vi "FPGA Combined SAR and DSA.vi"() -> ()   [LabVIEW 2025]
uses:
  <vilib>/Platform/TimedLoop/XDataNode/timing_clust.ctl
  <vilib>/Platform/TimedLoop/XDataNode/nitl_modes.ctl
  <vilib>/Platform/TimedLoop/XDataNode/wakeup.ctl
  <vilib>/LabVIEW Targets/FPGA/cRIO/shared/nicrio_ModuleControls/nicrio_cRIO-9234_DataRatesRing2.ctl
  <vilib>/rvi/Emulation/niFpgaGetClockAttributes.vi
  <vilib>/rvi/Emulation/niFpgaSctlEmulationGetInTimedLoop.vi
  <vilib>/rvi/Emulation/niFpgaEmulationReportErrorSimple.vi
  <vilib>/rvi/eio/common/nirviEmuTemplateMethod_errors.vi
  <vilib>/rvi/Emulation/niFpgaCriticalErrorInLSC.vi
  <vilib>/rvi/eio/common/nirviEmuTemplatePropertySet_noerrors.vi
  <vilib>/eio/utilities/niEioResolveVilibRelativePath.vi
  <vilib>/rvi/interface/RandomDataEmulation/niFpgaRandomDataHandleErrors.vi
  <vilib>/eio/EIONode/EIONode.xnode
  <vilib>/eio/EIOPropertyNode/EIOPropertyNode.xnode
  <vilib>/rvi/DataTransferAndStorage/Container/XNode/niFpgaContainer.xnode
  <vilib>/rvi/interface/RandomDataEmulation/nirviRandomDataFpgaReadWriteTemplate.vi
  <vilib>/platform/TimedLoop/XDataNode/XDataNode.xnode
  <vilib>/rvi/eio/common/nirviEmuTemplatePropertyGet_errors.vi
  <vilib>/rvi/eio/common/nirviEmuTemplatePropertyGet_noerrors.vi
  <vilib>/rvi/eio/common/nirviEmuTemplatePropertySet_errors.vi
  <vilib>/Platform/TimedLoop/XDataNode/XDNodeRunTimeDep.lvlib
panel:
  in  "stop Fast Digital":bool
  out "Mod2/DIO0":bool
  out "Mod2/DIO1":bool
  out "Mod2/DIO2":bool
  out "Mod2/DIO3":bool
  in  "stop Slow Digital":bool
  in  "Mod1/DO0":bool
  in  "Mod1/DO1":bool
  in  "Mod1/DO2":bool
  in  "Mod1/DO3":bool
  out "Combined Data":fxp<+/-,26,5>[](array[numeric])
  in  "stop Combined":bool
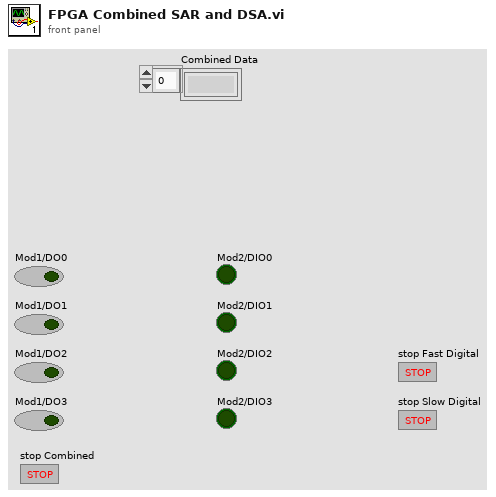
[diagram p1: front panel]
types:
  T1 = typedef "nicrio_cRIO-9234_DataRatesRing2.ctl" = u8
  T2 = typedef "XDNodeRunTimeDep.lvlib/timing_clust.ctl" = cluster{"Expected End [f-1]":u64, "Actual End [f-1]":u64, "Finished Late? [f-1]":bool, "Expected End [i-1]":u64, "Actual End [i-1]":u64, "Finished Late? [i-1]":bool, "Expected Start [i]":u64, "Actual Start [i]":u64, "Expected Start [f]":u64, "Actual Start [f]":u64, "Source Name":string, "Structure Name":string, "Period":i64, "Deadline":i64, "Offset":i64, "Start":i64, "Priority":i32, "Timeout":i32, "Mode":T3, "Wakeup Reason":T4, "Error":errorcluster, "Source Type":string, "Secondary Source Type":string, "Global End Time":u64, "Global Start Time":u64, "Frame Duration":u64, "Iteration Duration":u64, "Assigned CPU":i32, "I/O Scan Engine Mode":u32}
  T3 = typedef "XDNodeRunTimeDep.lvlib/nitl_modes.ctl" = enum32{"No Change", "Process missed periods, maintain original phase", "Discard missed periods, maintain original phase", "Process missed periods, ignore original phase", "Discard missed periods, ignore original phase"}
  T4 = typedef "XDNodeRunTimeDep.lvlib/wakeup.ctl" = enum32{"Normal", "Aborted", "Asynchronous wakeup", "Timing source error", "Timed loop error", "Timeout"}
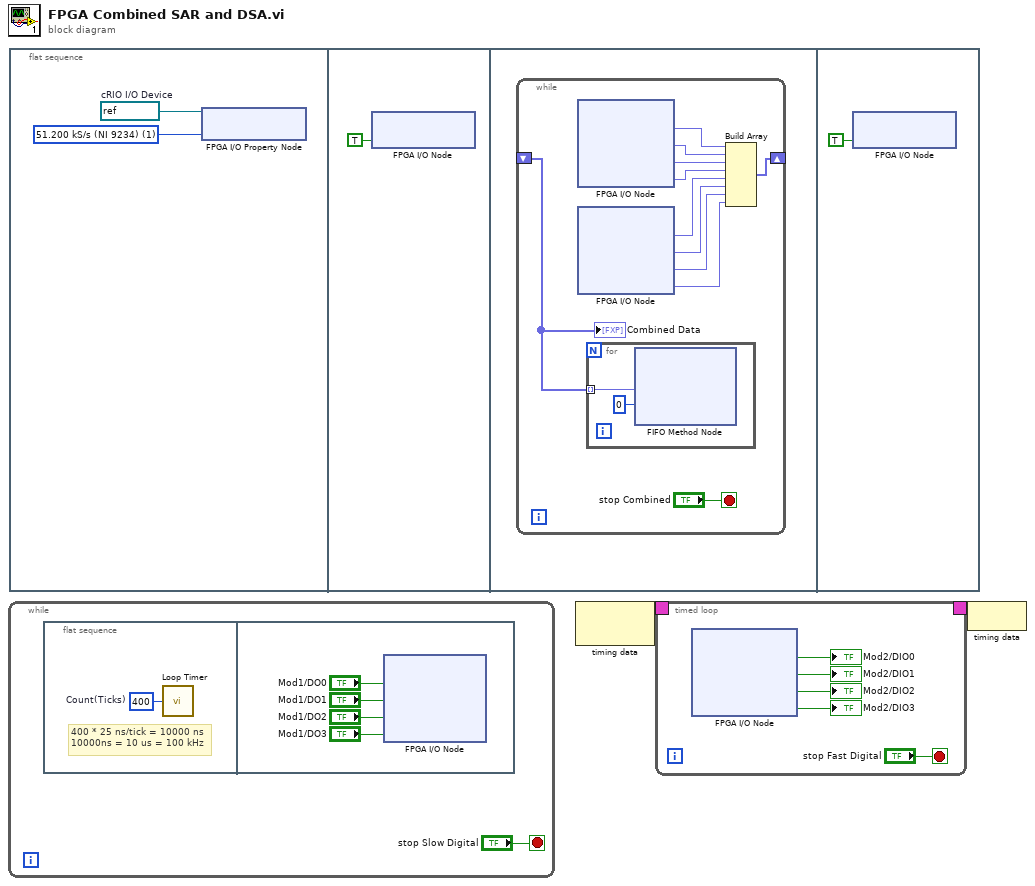
[diagram p0: block diagram]
diagram:
  n1 = while {
    stop <- "stop Slow Digital" stop-if-true
    n2 = flat-sequence {
      frame #0 {
        w4 = u32 400  # Count(Ticks)
        # "400 * 25 ns/tick = 10000 ns\n10000ns = 10 us = 100 kHz"
        n3 = call "Loop Timer"("Count(Ticks)"=w4) -> ()  [unwired: 1 out]
      }
      frame #1 {
        n4 = xnode "FPGA I/O Node"("Mod1/DO0"="Mod1/DO0", "Mod1/DO1"="Mod1/DO1", "Mod1/DO2"="Mod1/DO2", "Mod1/DO3"="Mod1/DO3") -> ()  [unwired: 4 in, 4 out]
      }
    }
  }
  n5 = flat-sequence {
    frame #0 {
      w9 = T1 1 items=["51.200 kS/s (NI 9234)"=1, "25.600 kS/s (NI 9234)"=2, "17.067 kS/s (NI 9234)"=3, "12.800 kS/s (NI 9234)"=4, "10.240 kS/s (NI 9234)"=5, "8.533 kS/s (NI 9234)"=6, "7.314 kS/s (NI 9234)"=7, "6.400 kS/s (NI 9234)"=8, "5.689 kS/s (NI 9234)"=9, "5.120 kS/s (NI 9234)"=10, "4.654 kS/s (NI 9234)"=11, "4.267 kS/s (NI 9234)"=12, "3.938 kS/s (NI 9234)"=13, "3.657 kS/s (NI 9234)"=14, "3.413 kS/s (NI 9234)"=15, "3.200 kS/s (NI 9234)"=16, "3.012 kS/s (NI 9234)"=17, "2.845 kS/s (NI 9234)"=18, "2.695 kS/s (NI 9234)"=19, "2.560 kS/s (NI 9234)"=20, "2.438 kS/s (NI 9234)"=21, "2.328 kS/s (NI 9234)"=22, "2.226 kS/s (NI 9234)"=23, "2.133 kS/s (NI 9234)"=24, "2.048 kS/s (NI 9234)"=25, "1.969 kS/s (NI 9234)"=26, "1.896 kS/s (NI 9234)"=27, "1.829 kS/s (NI 9234)"=28, "1.765 kS/s (NI 9234)"=29, "1.707 kS/s (NI 9234)"=30, "1.652 kS/s (NI 9234)"=31] ("Data Rate")
      w10 = refnum<k21> "Mod7"  # cRIO I/O Device
      n6 = xnode "FPGA I/O Property Node"("FPGA I/O In"=w10, "Data Rate"=w9) -> ()  [unwired: 1 out]
    }
    frame #1 {
      n7 = xnode "FPGA I/O Node"("Mod7/Start"=TRUE) -> ()  [unwired: 1 in, 1 out]
    }
    frame #2 {
      n8 = while {
        shift-right: [w21] -> _
        shift-left: _ -> [w12]
        stop <- "stop Combined" stop-if-true
        n9 = xnode "FPGA I/O Node"() -> ("Mod7/AI0"=w20:fxp<+/-,24,4>, "Mod7/AI1"=w19:fxp<+/-,24,4>, "Mod7/AI2"=w18:fxp<+/-,24,4>, "Mod7/AI3"=w17:fxp<+/-,24,4>)  [unwired: 4 in, 4 out]
        n10 = xnode "FPGA I/O Node"() -> ("Mod4/AI0"=w16:fxp<+/-,26,5>, "Mod4/AI1"=w15:fxp<+/-,26,5>, "Mod4/AI2"=w14:fxp<+/-,26,5>, "Mod4/AI3"=w13:fxp<+/-,26,5>)  [unwired: 4 in, 4 out]
        n11 = for {
          tunnel: w12 -> [w24] mode=indexing
          n12 = xnode ("FIFO Method Node")("Element"=w24, "Timeout"=0) -> ()  [unwired: 1 in, 2 out]
        }
        n13 = Build Array(w20, w19, w18, w17, w16, w15, w14, w13) -> (w21:fxp<+/-,26,5>[])
        "Combined Data" <- w12
      }
    }
    frame #3 {
      n14 = xnode "FPGA I/O Node"("Mod7/Stop"=TRUE ("Mod7/Start")) -> ()  [unwired: 1 in, 1 out]
    }
  }
  n15 = node-c288() -> (w2:T2)  [unwired: 1 in]
  n16 = timed-loop {
    timing: w2 -> [_]
    timing-out: [_] -> w1
    stop <- "stop Fast Digital" stop-if-true
    n17 = xnode "FPGA I/O Node"() -> ("Mod2/DIO0"=→"Mod2/DIO0":bool, "Mod2/DIO1"=→"Mod2/DIO1":bool, "Mod2/DIO2"=→"Mod2/DIO2":bool, "Mod2/DIO3"=→"Mod2/DIO3":bool)  [unwired: 4 in, 4 out]
  }
  n18 = node-c288(w1) -> ()
